vi "UML_Diagram.vi"() -> ()   [LabVIEW 2020]
uses:
  UMLClass/UMLClass.lvclass
  Collection/Collection.lvclass
  C:/Users/daal/OneDrive/LabVIEW/Picture2D/IDrawable/IDrawable.lvclass
  Point/Point.lvclass
  2DPictureControl/2DPictureControl.lvclass
  Line/Line.lvclass
  Triangle/Triangle.lvclass
  Pen/Pen.lvclass
  State_UML_Diagram.ctl
panel:
  in  "Sh:Point:y":i16(slide)=200
  in  "Sh:Point:x":i16(slide)=450 scale=0.0..1000.0
  in  "ID:Point:y":i16(slide)=10
  in  "ID:Point:x":i16(slide)=450 scale=0.0..1000.0
  out "2D Picture out":picture
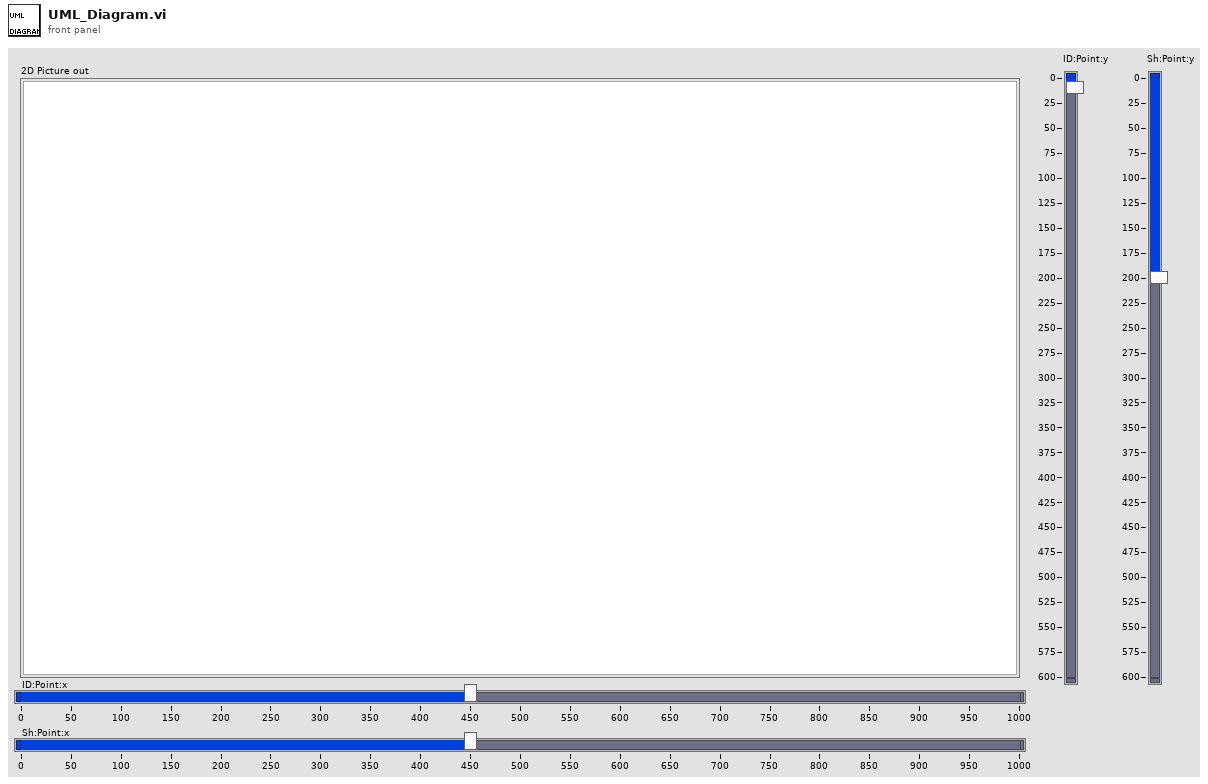
[diagram p1: front panel]
types:
  T1 = map{string, cluster{"Parent":string[], "Properties":string[], "Method":string[]}}
  T2 = typedef "Picture2D.lvlib/State_UML_Diagram.ctl" = enum16{"Get Class Hierarchy", "Draw Class"}
  T3 = enum32{"Solid", "Dash", "Dot", "DashDot", "DashDotDot"}
  T4 = cluster{"left":i16, "top":i16, "right":i16, "bottom":i16}
  T5 = cluster{"Parent":string[], "Properties":string[], "Method":string[]}[]
  T6 = cluster{"Parent":string[], "Properties":string[], "Method":string[]}
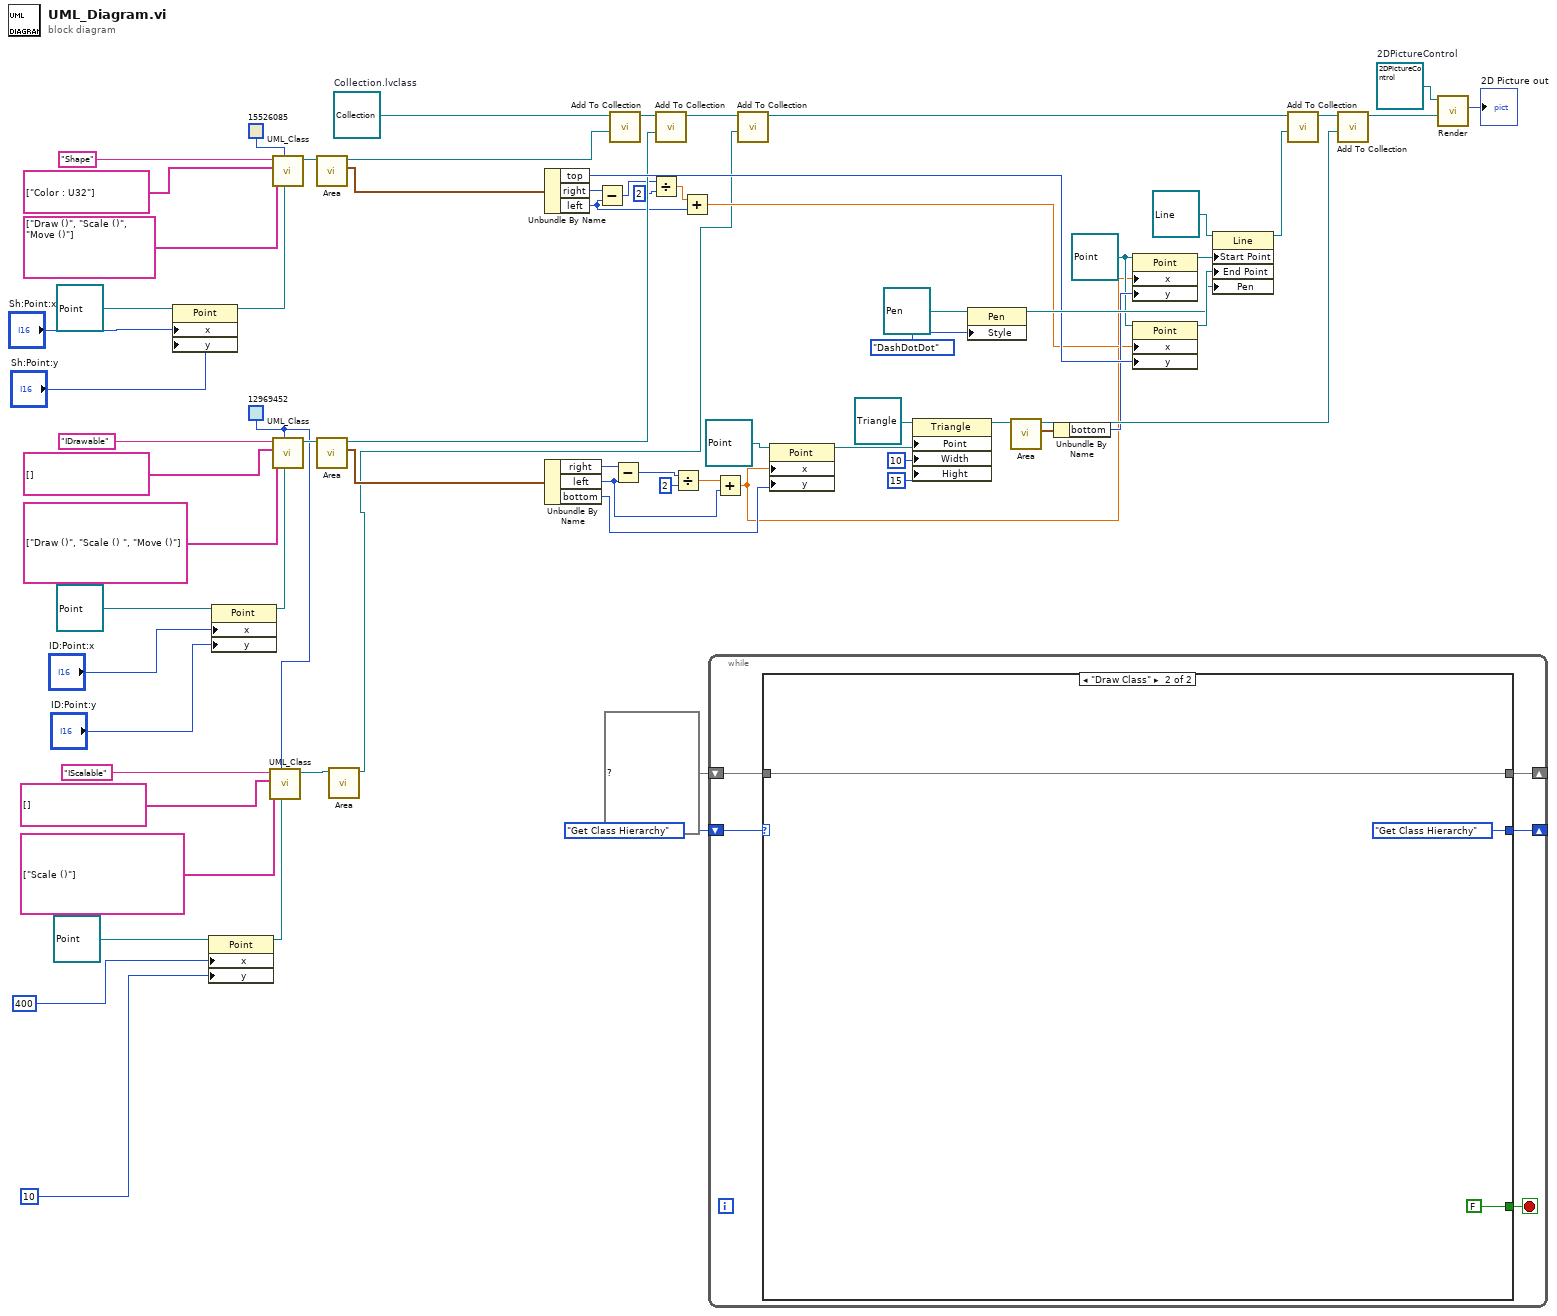
[diagram p0: block diagram]
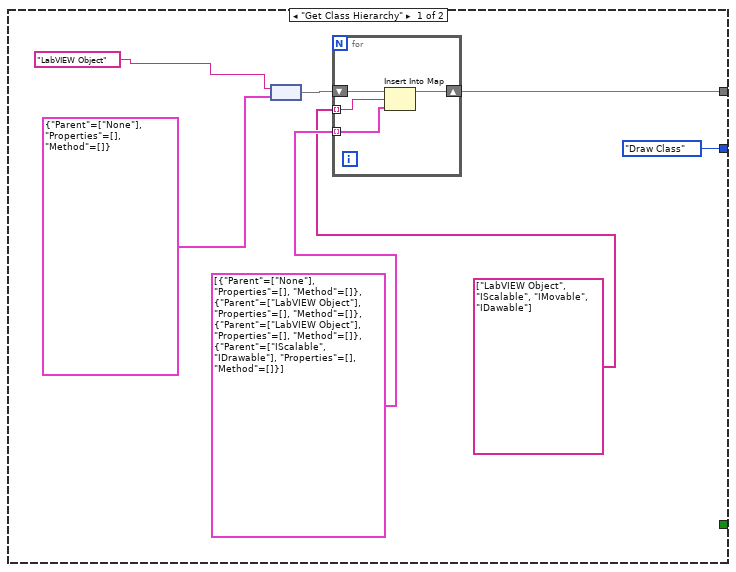
[diagram p2: hidden frame]
diagram:
  w9 = u32 12969452 ("Color")
  w19 = refnum<class "Point.lvclass"> refnum ("Point")
  w61 = refnum<class "2DPictureControl.lvclass"> refnum  # 2DPictureControl
  w72 = refnum<class "Collection.lvclass"> refnum  # Collection.lvclass
  n1 = property class="Point"(reference=refnum<class "Point.lvclass"> refnum ("Point"), "x"="Sh:Point:x", "y"="Sh:Point:y") -> (reference out=w57:refnum<class "Point.lvclass">)  [unwired: 1 in, 1 out]
  n2 = property class="Point"(reference=refnum<class "Point.lvclass"> refnum ("Point"), "x"=i16 400 ("ID:Point:x 2"), "y"=i16 10 ("ID:Point:y 2")) -> (reference out=w10:refnum<class "Point.lvclass">)  [unwired: 1 in, 1 out]
  n3 = property class="Point"(reference=refnum<class "Point.lvclass"> refnum ("Point"), "x"="ID:Point:x", "y"="ID:Point:y") -> (reference out=w64:refnum<class "Point.lvclass">)  [unwired: 1 in, 1 out]
  n4 = call "UML_Class.vi"("Point"=w10, "Color"=w9, "Methods"=string[] ["Scale ()"], "Properties"=string[] [], "Class Name"="IScalable") -> ("Collection out"=w8:refnum<class "Collection.lvclass">)  [unwired: 4 in, 2 out]
  n5 = call "UML_Class.vi"("Point"=w57, "Color"=u32 15526085, "Methods"=string[] ["Draw ()", "Scale ()", "Move ()"], "Properties"=string[] ["Color : U32"], "Class Name"="Shape") -> ("Collection out"=w42:refnum<class "Collection.lvclass">)  [unwired: 4 in, 2 out]
  n6 = call "UML_Class.vi"("Point"=w64, "Color"=w9, "Methods"=string[] ["Draw ()", "Scale () ", "Move ()"], "Properties"=string[] [], "Class Name"="IDrawable") -> ("Collection out"=w37:refnum<class "Collection.lvclass">)  [unwired: 4 in, 2 out]
  n7 = call-dynamic "Area.vi"("Collection in"=w42) -> ("Area"=w40:T4, "Collection out"=w41:refnum<class "Collection.lvclass">)  [unwired: 8 in, 1 out]
  n8 = call-dynamic "Area.vi"("Collection in"=w37) -> ("Area"=w35:T4, "Collection out"=w36:refnum<class "Collection.lvclass">)  [unwired: 8 in, 1 out]
  n9 = call-dynamic "Area.vi"("Collection in"=w8) -> ("Collection out"=w5:refnum<class "Collection.lvclass">)  [unwired: 8 in, 2 out]
  n10 = Unbundle By Name(w40) -> ("top"=w39:i16, "right"=w24:i16, "left"=w23:i16)
  n11 = Unbundle By Name(w35) -> ("right"=w31:i16, "left"=w27:i16, "bottom"=w18:i16)
  n12 = Subtract(x=w24, y=w23) -> (x-y=w22:i16)
  n13 = call-dynamic "Add To Collection.vi"("IDrawable"=w41, "Collection in"=w72) -> ("Collection out"=w55:refnum<class "Collection.lvclass">)  [unwired: 8 in, 1 out]
  n14 = Subtract(x=w31, y=w27) -> (x-y=w30:i16)
  n15 = Divide(x=w22, y=i16 2) -> (x/y=w25:dbl)
  n16 = call-dynamic "Add To Collection.vi"("IDrawable"=w36, "Collection in"=w55) -> ("Collection out"=w7:refnum<class "Collection.lvclass">)  [unwired: 8 in, 1 out]
  n17 = Divide(x=w30, y=i16 2) -> (x/y=w28:dbl)
  n18 = Add(x=w25, y=w23) -> (x+y=w17:dbl)
  n19 = while {
    shift-right: [w74] -> _
    shift-left: State_UML_Diagram."Get Class Hierarchy" -> [w77]
    shift-right: [w76] -> _
    shift-left: T1 {} ("map") -> [w75]
    stop <- w73 stop-if-true
    n20 = case shown="\"Draw Class\"" w77 {
      tunnel: [w79 w91] -> w76
      tunnel: w75 -> [_ w91]
      tunnel: [State_UML_Diagram."Draw Class" State_UML_Diagram."Get Class Hierarchy"] -> w74
      tunnel: [_ FALSE] -> w73
      frame "Get Class Hierarchy" {
        n21 = node("LabVIEW Object", T6 {"Parent"=["None"], "Properties"=[], "Method"=[]}) -> (w83:T1)
        n22 = for {
          shift-right: [w87] -> w79
          shift-left: w83 -> [w88]
          tunnel: T5 [{"Parent"=["None"], "Properties"=[], "Method"=[]}, {"Parent"=["LabVIEW Object"], "Properties"=[], "Method"=[]}, {"Parent"=["LabVIEW Object"], "Properties"=[], "Method"=[]}, {"Parent"=["IScalable", "IDrawable"], "Properties"=[], "Method"=[]}] -> [w86] mode=indexing
          tunnel: string[] ["LabVIEW Object", "IScalable", "IMovable", "IDawable"] -> [w85] mode=indexing
          n23 = Insert Into Map(map in=w88, key=w85, value=w86) -> (map out=w87:T1)  [unwired: 2 out]
        }
      }
      frame "Draw Class" {
      }
    }
  }
  n24 = Add(x=w28, y=w27) -> (x+y=w16:dbl)
  n25 = call-dynamic "Add To Collection.vi"("IDrawable"=w5, "Collection in"=w7) -> ("Collection out"=w6:refnum<class "Collection.lvclass">)  [unwired: 8 in, 1 out]
  n26 = property class="Point"(reference=refnum<class "Point.lvclass"> refnum ("Point"), "x"=w16, "y"=w18) -> (reference out=w43:refnum<class "Point.lvclass">)  [unwired: 1 in, 1 out]
  n27 = property class="Triangle"(reference=refnum<class "Triangle.lvclass"> refnum ("Triangle"), "Point"=w43, "Width"=i16 10, "Hight"=i16 15) -> (reference out=w34:refnum<class "Triangle.lvclass">)  [unwired: 1 in, 1 out]
  n28 = property class="Pen"(reference=refnum<class "Pen.lvclass"> refnum ("Pen"), "Style"=T3."DashDotDot" ("Pen:Style")) -> (reference out=w46:refnum<class "Pen.lvclass">)  [unwired: 1 in, 1 out]
  n29 = call-dynamic "Area.vi"("Triangle in"=w34) -> ("rect"=w21:T4, "Triangle out"=w33:refnum<class "Triangle.lvclass">)  [unwired: 8 in, 1 out]
  n30 = Unbundle By Name(w21) -> ("bottom"=w20:i16)
  n31 = property class="Point"(reference=w19, "x"=w16, "y"=w20) -> (reference out=w44:refnum<class "Point.lvclass">)  [unwired: 1 in, 1 out]
  n32 = property class="Point"(reference=w19, "x"=w17, "y"=w39) -> (reference out=w50:refnum<class "Point.lvclass">)  [unwired: 1 in, 1 out]
  n33 = property class="Line"(reference=refnum<class "Line.lvclass"> refnum ("Line"), "Start Point"=w44, "End Point"=w50, "Pen"=w46) -> (reference out=w38:refnum<class "Line.lvclass">)  [unwired: 1 in, 1 out]
  n34 = call-dynamic "Add To Collection.vi"("IDrawable"=w38, "Collection in"=w6) -> ("Collection out"=w52:refnum<class "Collection.lvclass">)  [unwired: 8 in, 1 out]
  n35 = call-dynamic "Add To Collection.vi"("IDrawable"=w33, "Collection in"=w52) -> ("Collection out"=w59:refnum<class "Collection.lvclass">)  [unwired: 8 in, 1 out]
  n36 = call-dynamic "Render.vi"("IDrawable"=w59, "2DPictureControl in"=w61) -> ("2D Picture out"=→"2D Picture out":picture)  [unwired: 7 in, 2 out]
